vi "CS_Prepare_TDMS.vi"(8 "error in (no error)":errorcluster, 11 "Save path":path) -> (0 "error out":errorcluster, 3 "Refnum out":refnum<k34>)   [LabVIEW 2018, in "Tracker.lvlib"]
uses:
  Tracker.lvlib
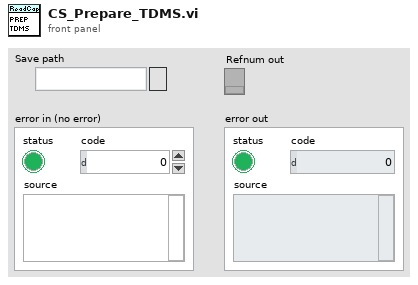
[diagram p1: front panel]
types:
  T1 = enum16{"open", "open or create", "create or replace", "create", "open (read-only)"}
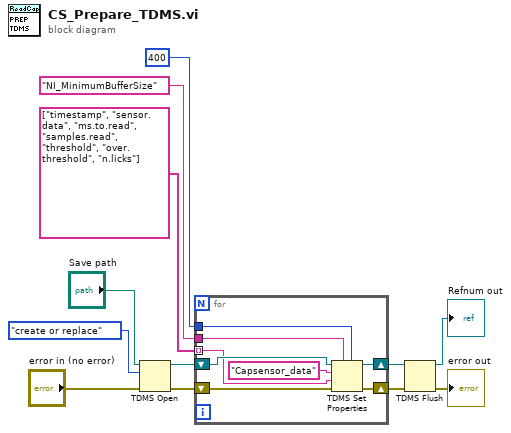
[diagram p0: block diagram]
diagram:
  n1 = TDMS Open(8:"error in (no error)", 10:T1."create or replace" ("operation (0:open)"), 11:"Save path") -> (0:w7:errorcluster, 3:w6:refnum<k34>)  [unwired: 4 in]
  n2 = for {
    tunnel: string[] ["timestamp", "sensor.data", "ms.to.read", "samples.read", "threshold", "over.threshold", "n.licks"] ("Columns Names") -> [w17] mode=indexing
    tunnel: "NI_MinimumBufferSize" -> [w16]
    tunnel: 400 ("Buffer size, samples") -> [w15]
    shift-right: [w14] -> w9
    shift-left: w6 -> [w20]
    shift-right: [w13] -> w10
    shift-left: w7 -> [w19]
    n3 = TDMS Set Properties(5:w15, 7:w16, 8:w19, 9:w17, 10:"Capsensor_data" ("group name"), 11:w20) -> (0:w13:errorcluster, 3:w14:refnum<k34>)  [unwired: 2 out]
  }
  n4 = TDMS Flush(4:w10, 7:w9) -> (0:→"error out":errorcluster, 3:→"Refnum out":refnum<k34>)
